vi "TCP Write Data.vi"(4 "error in (no error)":errorcluster, 5 "timeout ms (25000)":i32=25000, 6 "Flattened Data":string, 7 "connection ID":refnum<k5>) -> (0 "error out":errorcluster, 2 "bytes written":i32, 3 "dup connection ID":refnum<k5>)   [LabVIEW 2011]
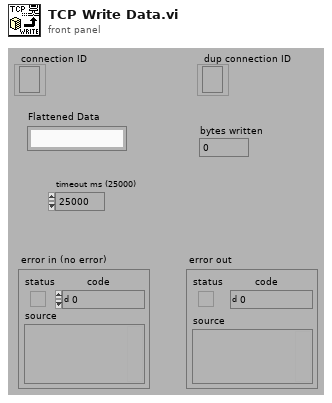
[diagram p1: front panel]
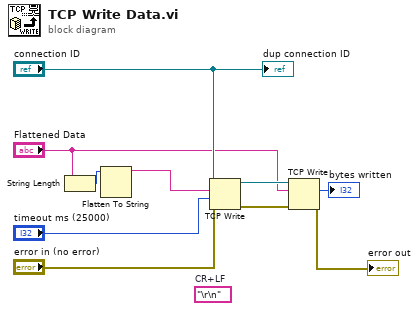
[diagram p0: block diagram]
diagram:
  (unwired) "\r\n"  # CR+LF
  n1 = String Length(string="Flattened Data") -> (length=w4:i32)
  n2 = Flatten To String(anything=w4) -> (data string=w2:string)  [unwired: 1 in, 4 out]
  n3 = TCP Write(connection ID="connection ID", data in=w2, error in (no error)="error in (no error)", 9:"timeout ms (25000)") -> (connection ID out=w10:refnum<k5>, error out=w9:errorcluster)  [unwired: 1 out]
  n4 = TCP Write(connection ID=w10, data in="Flattened Data", error in (no error)=w9) -> (bytes written=→"bytes written":i32, error out=→"error out":errorcluster)  [unwired: 2 out]
  "dup connection ID" <- "connection ID"
